vi "Tree Manager.vi"(7 "Mode":T4, 10 "Settings In":T1={"Step Values"=[], "Only Execute When Test Running"=TRUE, "Reset Sequence When Test Starts"=TRUE, "Current Sequence ID"=0, "Total Iterations"=0, "Last Timestamp"=0.0, "Number of Sequence Steps"=0, "Num of Analog Channels"=0, "Num of Digital Channels"=0, "Delay Before Starting Sequence"=0.0, "Changed"=FALSE}, 11 "Init Refs":T3) -> (3 "Settings Out":T1={"Step Values"=[], "Only Execute When Test Running"=TRUE, "Reset Sequence When Test Starts"=TRUE, "Current Sequence ID"=0, "Total Iterations"=0, "Last Timestamp"=0.0, "Number of Sequence Steps"=0, "Num of Analog Channels"=0, "Num of Digital Channels"=0, "Delay Before Starting Sequence"=0.0, "Changed"=FALSE})   [LabVIEW 2020, in "Sequencer with Output Values.lvlib" / "Sequencer with Output Values.lvclass"]
uses:
  Sequencer with Output Values.lvclass
  Tree Manager Mode.ctl
  Control Refs.ctl
  Params.ctl
  Step Settings.ctl
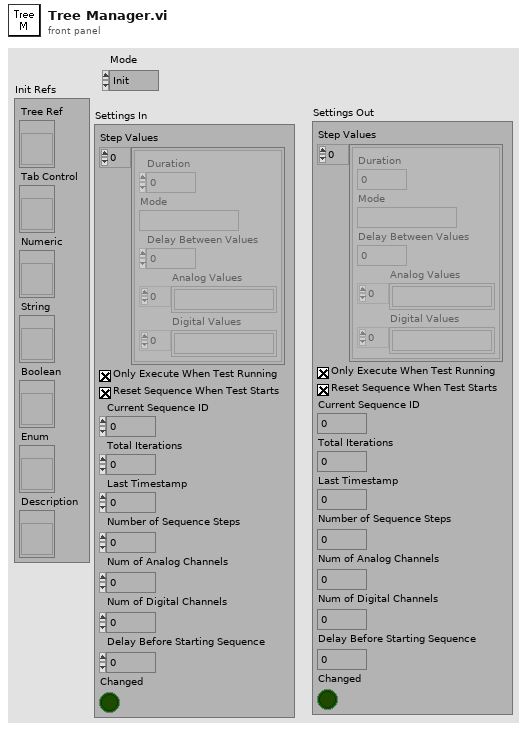
[diagram p1: front panel]
types:
  T1 = typedef "Sequencer with Output Values.lvlib/Sequencer with Output Values.lvclass/Params.ctl" = cluster{"Step Values":T2[], "Only Execute When Test Running":bool, "Reset Sequence When Test Starts":bool, "Current Sequence ID":u32, "Total Iterations":u32, "Last Timestamp":dbl, "Number of Sequence Steps":i32, "Num of Analog Channels":i32, "Num of Digital Channels":i32, "Delay Before Starting Sequence":dbl, "Changed":bool}
  T2 = typedef "Sequencer with Output Values.lvlib/Sequencer with Output Values.lvclass/Step Settings.ctl" = cluster{"Duration":dbl, "Mode":string, "Delay Between Values":dbl, "Analog Values":string[], "Digital Values":string[]}
  T3 = typedef "Sequencer with Output Values.lvlib/Sequencer with Output Values.lvclass/Control Refs.ctl" = cluster{"Tree Ref":refnum<vi>, "Tab Control":refnum<vi>, "Numeric":refnum<vi>, "String":refnum<vi>, "Boolean":refnum<vi>, "Enum":refnum<vi>, "Description":refnum<vi>}
  T4 = typedef "Sequencer with Output Values.lvlib/Sequencer with Output Values.lvclass/Tree Manager Mode.ctl" = enum16{"Init", "Tree Change", "Value Change"}
  T5 = typedef "Sequencer with Output Values.lvlib/Sequencer with Output Values.lvclass/Tree Item Settings.ctl" = cluster{"Indent Level":i32, "Data Type":T6, "Numeric Range":cluster{"Min":dbl, "Max":dbl, "Inc":dbl}, "Enum Values":string[], "Default Value":string}
  T6 = typedef "Sequencer with Output Values.lvlib/Sequencer with Output Values.lvclass/Data Type.ctl" = i16
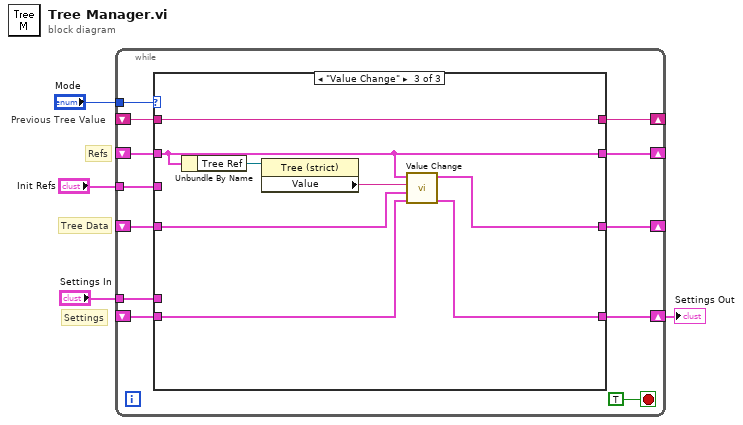
[diagram p0: block diagram]
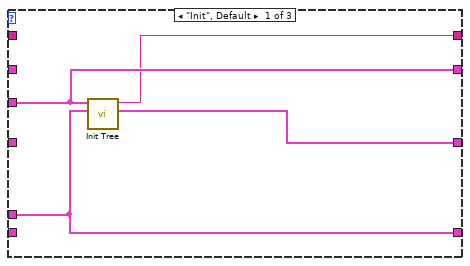
[diagram p2: hidden frame]
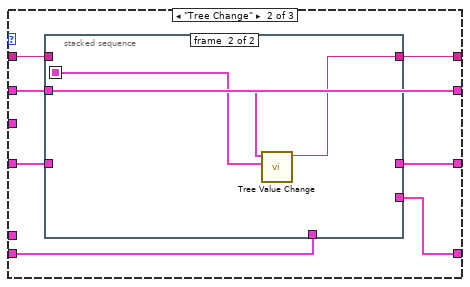
[diagram p3: hidden frame]
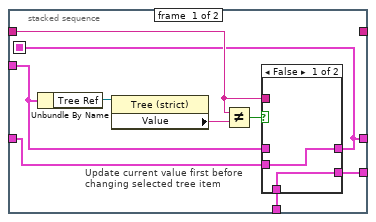
[diagram p4: hidden frame]
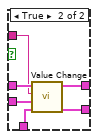
[diagram p5: hidden frame]
diagram:
  # "Previous Tree Value"
  # "Tree Data"
  # "Settings"
  # "Refs"
  n1 = while {
    tunnel: "Mode" -> [w16]
    tunnel: "Init Refs" -> [w15]
    tunnel: "Settings In" -> [w13]
    shift-right: [w12] -> _
    shift-left: _ -> [w11]
    shift-right: [w10] -> w1
    shift-left: _ -> [w9]
    shift-right: [w8] -> _
    shift-left: _ -> [w7]
    shift-right: [w6] -> _
    shift-left: _ -> [w5]
    stop <- TRUE stop-if-true
    n2 = case shown="\"Value Change\"" w16 {
      tunnel: w15 -> [w20 _ _]
      tunnel: w13 -> [w18 _ _]
      tunnel: [w20 w26 w54] -> w12
      tunnel: w11 -> [_ w26 w54]
      tunnel: [w18 w22 w48] -> w10
      tunnel: w9 -> [_ w23 w50]
      tunnel: [w19 w21 w49] -> w8
      tunnel: w7 -> [_ w27 w51]
      tunnel: [w17 w25 w55] -> w6
      tunnel: w5 -> [_ w24 w55]
      frame "Init", Default {
        n3 = call "Init Tree.vi"("Settings In"=w18, "Init Refs"=w20) -> ("Tree Data"=w19:cluster{string[], T5[]}, "Selected Tag"=w17:string)  [unwired: 8 in]
      }
      frame "Tree Change" {
        n4 = stacked-sequence {
          seq-local: [w28 _] -> [_ w45]
          tunnel: w27 -> [w31 _]
          tunnel: w26 -> [w35 w47]
          tunnel: [_ w46] -> w25
          tunnel: w24 -> [w32 _]
          tunnel: w23 -> [w30 _]
          tunnel: [w29 _] -> w22
          tunnel: [w28 _] -> w21
          frame #0 {
            # "Update current value first before changing selected tree item"
            n5 = Unbundle By Name(w35) -> ("Tree Ref"=w36:refnum<vi>)
            n6 = property class="Tree (strict)"(reference=w36) -> ("Value"=w34:string)  [unwired: 1 in, 2 out]
            n7 = Not Equal?(x=w32, y=w34) -> (x != y?=w33:bool)
            n8 = case shown="False" w33 {
              tunnel: w35 -> [_ w44]
              tunnel: w32 -> [_ w43]
              tunnel: w31 -> [w38 w42]
              tunnel: w30 -> [w37 w41]
              tunnel: [w38 w40] -> w28
              tunnel: [w37 w39] -> w29
              frame False {
              }
              frame True {
                n9 = call "Value Change.vi"("Settings In"=w41, "Tree Data"=w42, "Tree Tag"=w43, "Init Refs"=w44) -> ("Settings Out"=w39:T1, "Tree Data out"=w40:cluster{"Tag":string[], "Settings":T5[]})  [unwired: 6 in]
              }
            }
          }
          frame #1 {
            n10 = call "Tree Value Change.vi"("Tree Data"=w45, "Init Refs"=w47) -> ("Value"=w46:string)  [unwired: 9 in]
          }
        }
      }
      frame "Value Change" {
        n11 = Unbundle By Name(w54) -> ("Tree Ref"=w53:refnum<vi>)
        n12 = property class="Tree (strict)"(reference=w53) -> ("Value"=w52:string)  [unwired: 1 in, 2 out]
        n13 = call "Value Change.vi"("Settings In"=w50, "Tree Data"=w51, "Tree Tag"=w52, "Init Refs"=w54) -> ("Settings Out"=w48:T1, "Tree Data out"=w49:cluster{"Tag":string[], "Settings":T5[]})  [unwired: 6 in]
      }
    }
  }
  "Settings Out" <- w1
